vi "test_00_temp.vi"() -> ()   [LabVIEW 2015]
uses:
  lv-unit-conversion/public/advanced/save_dictinoary_json.vi
  lv-unit-conversion/lv-unit-conversion.lvlib
panel:
  out "value out":dbl
  in  "value in":dbl
  in  "from_unit":string="m"
  in  "to_unit":string="in"
  out "data_set":variant
  out "error out":errorcluster
  in  "error in (no error)":errorcluster
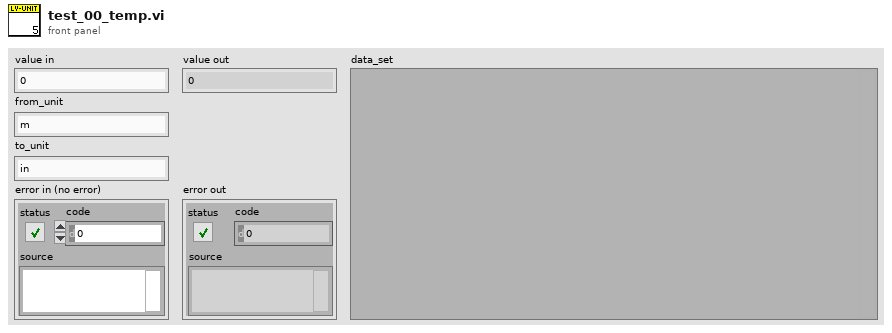
[diagram p1: front panel]
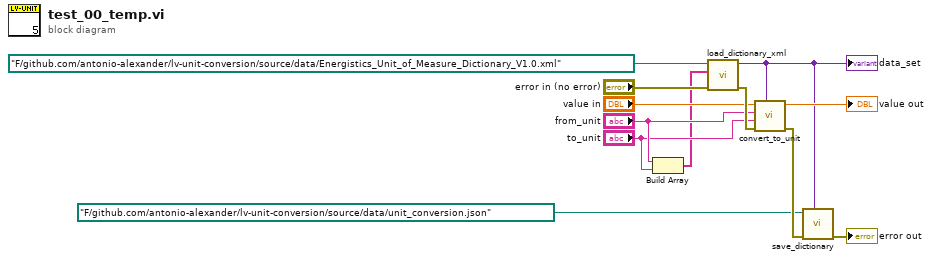
[diagram p0: block diagram]
diagram:
  n1 = Build Array("from_unit", "to_unit") -> (w1:string[])
  n2 = call "load_dictionary_xml.vi"("error in (no error)"="error in (no error)", "symbols []"=w1, "xml_path"=path "F:/github.com/antonio-alexander/lv-unit-conversion/source/data/Energistics_Unit_of_Measure_Dictionary_V1.0.xml" ("XML File Path")) -> ("error out"=w12:errorcluster, "unit_dictionary"=w2:variant)  [unwired: 7 in]
  "data_set" <- w2
  n3 = call "convert_to_unit.vi"("unit_dictionary"=w2, "error in (no error)"=w12, "unit_to"="to_unit", "unit_from"="from_unit", "value in"="value in") -> ("error out"=w5:errorcluster, "value out"=→"value out":dbl)  [unwired: 5 in]
  n4 = call-poly "save_dictionary.vi"("unit_dictionary"=w2, "error in (no error)"=w5, "json_path"=path "F:/github.com/antonio-alexander/lv-unit-conversion/source/data/unit_conversion.json") -> ("error out"=→"error out":errorcluster)  [unwired: 8 in]
